vi "Initialise Process.vi"(7 "Process":refnum<vi>, 8 "error in (no error)":errorcluster, 9 "Parameters":string[](array[string]), 10 "Steps (Initialise)":string[](array[string])=["Initialise"], 11 "Actor in":refnum<class "Actor.lvclass">) -> (0 "error out":errorcluster, 3 "Actor out":refnum<class "Actor.lvclass">)   [LabVIEW 2015, in "Actor.lvclass"]
uses:
  Actor.lvclass
  Actor.lvclass/Actor.ctl
  Sequencer/Sequencer.lvclass
  Utility/Utility.lvlib
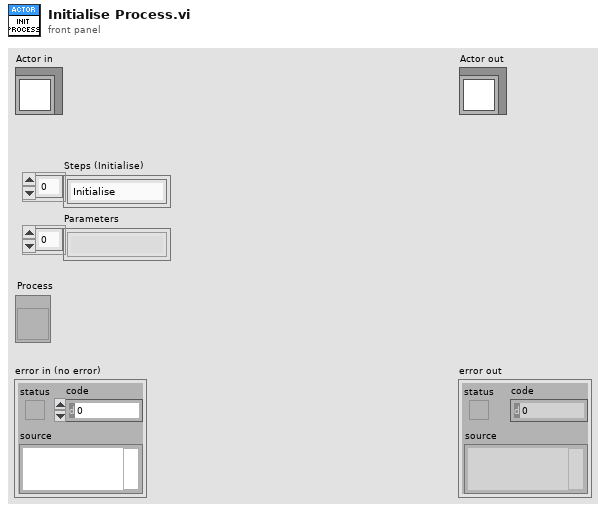
[diagram p1: front panel]
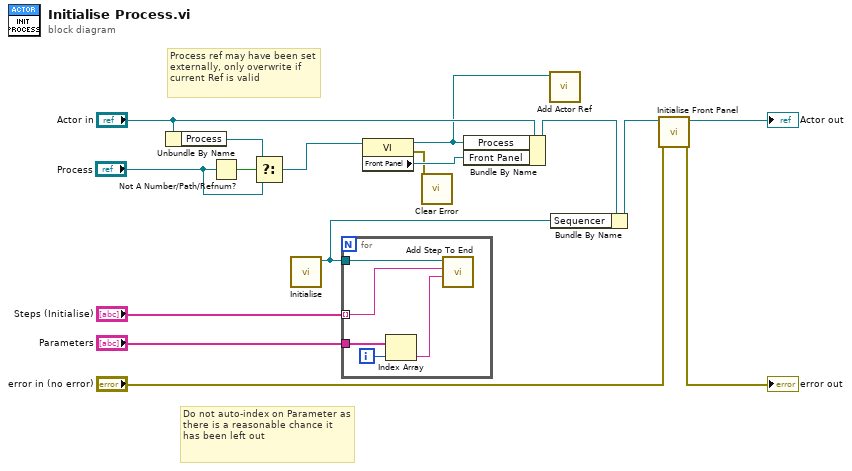
[diagram p0: block diagram]
diagram:
  # "Process ref may have been set externally, only overwrite if current Ref is valid"
  # "Do not auto-index on Parameter as there is a reasonable chance it has been left out"
  n1 = Unbundle By Name("Actor in") -> ("Process"=w6:refnum<vi>)
  n2 = Not A Number/Path/Refnum?(number/path/refnum="Process") -> (NaN/Path/Refnum?=w8:bool)
  n3 = Select(t=w6, s=w8, f="Process") -> (s? t:f=w4:refnum<vi>)
  n4 = call "Initialise.vi"() -> ("Sequencer out"=w5:refnum<class "Sequencer.lvclass">)  [unwired: 10 in, 1 out]
  n5 = for {
    tunnel: "Steps (Initialise)" -> [w20] mode=indexing
    tunnel: "Parameters" -> [w19]
    tunnel: w5 -> [w21]
    i -> [w18]
    n6 = Index Array(array=w19, index=w18) -> (element=w17:string)
    n7 = call "Add Step To End.vi"("Parameter"=w17, "Step Name"=w20, "Sequencer in"=w21) -> ()  [unwired: 8 in, 1 out]
  }
  n8 = property class="VI"(reference=w4) -> (reference out=w3:refnum<vi>, error out=w1:errorcluster, "Front Panel"=w2:refnum<vi>)  [unwired: 1 in]
  n9 = call "Clear Error.vi"("error in (no error)"=w1) -> ()  [unwired: 1 out]
  n10 = Bundle By Name(cluster="Actor in", "Process"=w3, "Front Panel"=w2) -> (w7:refnum<class "Actor.lvclass">)
  n11 = call "Add Actor Ref.vi"("VI Refnum In"=w3) -> ()  [unwired: 11 in]
  n12 = Bundle By Name(cluster=w7, "Sequencer"=w5) -> (w9:refnum<class "Actor.lvclass">)
  n13 = call-dynamic "Initialise Front Panel.vi"("error in (no error)"="error in (no error)", "Actor in"=w9) -> ("error out"=→"error out":errorcluster, "Actor out"=→"Actor out":refnum<class "Actor.lvclass">)  [unwired: 8 in]
